vi "Custom_FPGA_Target_Host_Example.vi"() -> ()   [LabVIEW 2024]
uses:
  <vilib>/FPGAPlugInAG/Dynamic/niLvFpga_Download_Dynamic.vi
  <vilib>/FPGAPlugInAG/Dynamic/niLvFpga_Run_Dynamic.vi
  <vilib>/FPGAPlugInAG/Dynamic/niLvFpga_Close_Dynamic.vi
  <vilib>/rvi/interface/nirviMethod/nirviMethod.xnode
  <vilib>/rvi/interface/nirviCloseFPGA/nirviCloseFPGA.xnode
panel:
  out "error out":errorcluster
  in  "Write Value":u32
  out "Read Value":u32
  out "Read Error":errorcluster
  out "Write Error":errorcluster
  in  "Write Offset":u32
  in  "Read Offset":u32
  in  "Write Register":bool
  in  "Read Register":bool
  in  "stop":bool
  out "Loop Count":i32
  in  "Bitfile path":path
  in  "Device address":string
  # "This is a simple example to demonstrate reading and writing \nFPGA HDL registers from the host PC.\n\nInstructions:\n1) Set the device address and bitfile path\n\n2) Run the VI\n\n3) Set the Read Offset to the offset of the register you want to read\n    Click Read Register\n\n4) Set the Write Offset to the offset of the register you want to write\n    Set the Write Value\n    Click Write Register"
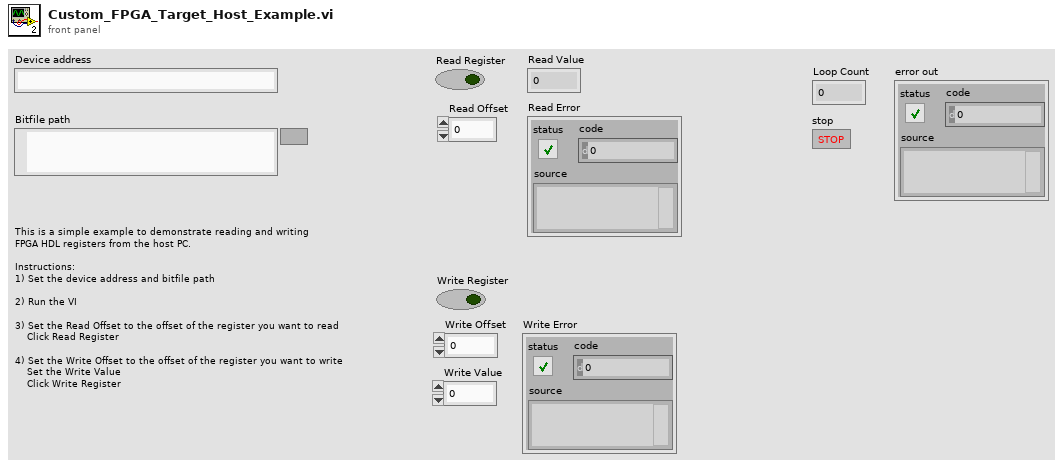
[diagram p1: front panel]
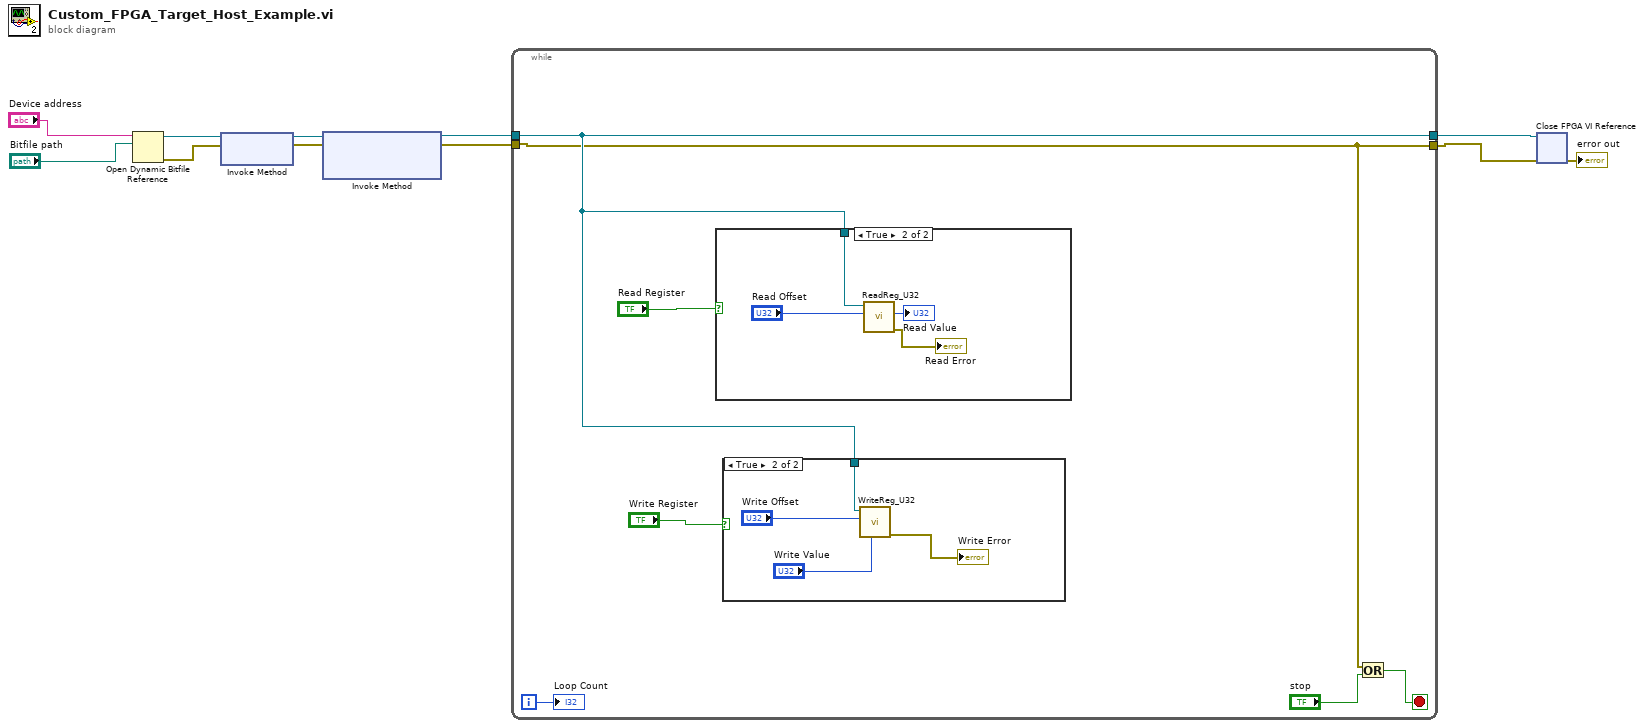
[diagram p0: block diagram]
diagram:
  n1 = Open Dynamic Bitfile Reference(0:"Device address", 1:"Bitfile path") -> (5:w9:refnum<k20>, 8:w8:errorcluster)  [unwired: 3 in]
  n2 = xnode "Invoke Method"("FPGA VI Reference In"=w9, "error in"=w8) -> ("FPGA VI Reference Out"=w7:refnum<k20>, "error out"=w6:errorcluster)
  n3 = xnode "Invoke Method"("FPGA VI Reference In"=w7, "error in"=w6) -> ("FPGA VI Reference Out"=w5:refnum<k20>, "error out"=w4:errorcluster)  [unwired: 1 in]
  n4 = while {
    tunnel: w5 -> [w15]
    tunnel: w4 -> [w14]
    tunnel: [w15] -> w3
    tunnel: [w14] -> w2
    i -> [w18]
    stop <- w12 stop-if-true
    n5 = case shown="True" "Read Register" {
      tunnel: w15 -> [_ w26]
      frame False {
      }
      frame True {
        n6 = call "ReadReg_U32.vi"("Offset"="Read Offset", "FPGA VI Reference In"=w26) -> ("error out"=→"Read Error":errorcluster, "value"=→"Read Value":u32)  [unwired: 7 in, 1 out]
      }
    }
    n7 = case shown="True" "Write Register" {
      tunnel: w15 -> [_ w22]
      frame False {
      }
      frame True {
        n8 = call "WriteReg_U32.vi"("Value"="Write Value", "Offset"="Write Offset", "FPGA VI Reference In"=w22) -> ("error out"=→"Write Error":errorcluster)  [unwired: 6 in, 1 out]
      }
    }
    n9 = Or(x=w14, y="stop") -> (x .or. y?=w12:bool)
    "Loop Count" <- w18
  }
  n10 = xnode "Close FPGA VI Reference"("FPGA VI Reference In"=w3, "error in"=w2) -> ("error out"=→"error out":errorcluster)
